vi "Expire Stale Hosts.vi"(0 "Known Hosts in":T1[](array[typedef]), 9 "timeout (s)":dbl=10.0) -> (4 "Known hosts out":T1[](array[typedef]), 8 "Expired":T1[](array[typedef]))   [LabVIEW 2020, in "epl-network.lvlib"]
uses:
  epl-network.lvlib
  Discovered Host.ctl
  Public/Discovery/Typedefs/Server Beacon.ctl
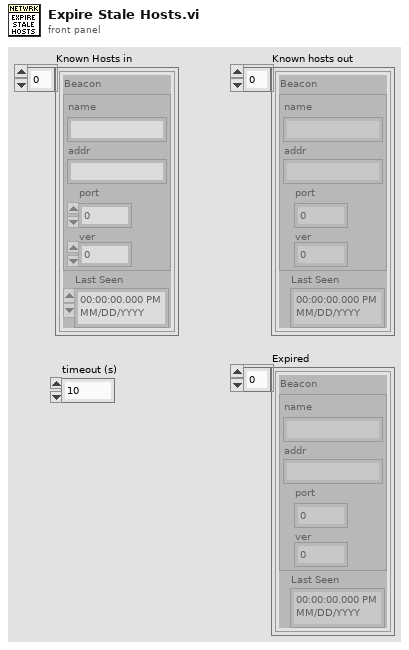
[diagram p1: front panel]
types:
  T1 = typedef "epl-network.lvlib/Discovered Host.ctl" = cluster{"Beacon":T2, "Last Seen":timestamp}
  T2 = typedef "epl-network.lvlib/Server Beacon.ctl" = cluster{"name":string, "addr":string, "port":u16, "ver":u16}
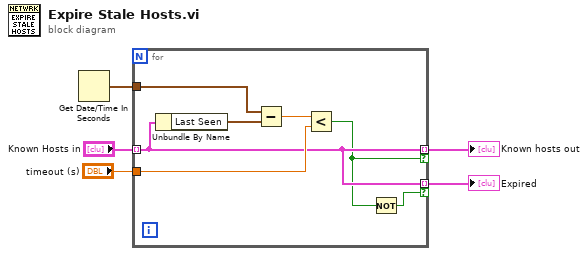
[diagram p0: block diagram]
diagram:
  n1 = Get Date/Time In Seconds() -> (seconds since 1Jan1904=w4:timestamp)
  n2 = for {
    tunnel: "Known Hosts in" -> [w8] mode=indexing
    tunnel: w4 -> [w12]
    tunnel: "timeout (s)" -> [w9]
    tunnel: [w8] -> w2 mode=indexing if=w6
    tunnel: [w8] -> w1 mode=indexing if=w7
    n3 = Unbundle By Name(w8) -> ("Last Seen"=w11:timestamp)
    n4 = Subtract(x=w12, y=w11) -> (x-y=w10:dbl)
    n5 = Less?(x=w10, y=w9) -> (x < y?=w6:bool)
    n6 = Not(x=w6) -> (.not. x?=w7:bool)
  }
  "Known hosts out" <- w2
  "Expired" <- w1
